vi "write_section_analysis_parameters_to_results_file.vi"(8 "Error In":errorcluster, 11 "Section Parameters":T1) -> (0 "Error Out":errorcluster)   [LabVIEW 2019]
uses:
  section_parameters_cluster_typedef.ctl
  sections_method_enum_typedef.ctl
  sections_edge_mode_enum_typedef.ctl
  sections_roi_size_enum_typedef.ctl
  xi_angles_enum_typedef.ctl
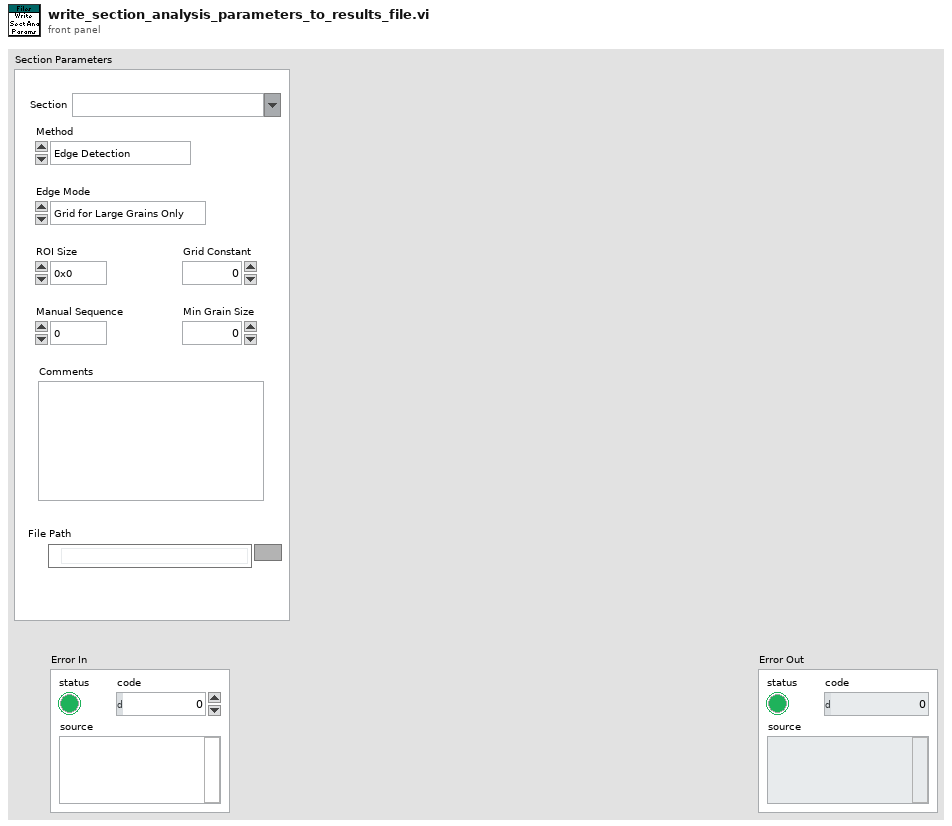
[diagram p1: front panel]
types:
  T1 = typedef "section_parameters_cluster_typedef.ctl" = cluster{"Section":string, "Method":T2, "Edge Mode":T3, "ROI Size":T4, "Manual Sequence":T5, "Grid Constant":i32, "Min Grain Size":dbl, "Comments":string, "File Path":path}
  T2 = typedef "sections_method_enum_typedef.ctl" = enum16{"Edge Detection", "Grid Only", "Manual Selection", "Existing Edges"}
  T3 = typedef "sections_edge_mode_enum_typedef.ctl" = enum16{"Grid for Large Grains Only", "Grid", "No Grid"}
  T4 = typedef "sections_roi_size_enum_typedef.ctl" = enum16{"0x0", "1x1", "2x2", "3x3", "4x4", "5x5", "6x6"}
  T5 = typedef "xi_angles_enum_typedef.ctl" = enum16{"0", "45"}
  T6 = typedef "writeable_section_parameters_cluster_typedef.ctl" = cluster{"Section":string, "Method":i32, "Edge Mode":i32, "Grid Constant":i32, "Manual Sequence":i32, "ROI Size":i32, "Min Grain Size":dbl, "Comments":string, "File Path":string}
  T7 = typedef "sample_results_cluster_typedef.ctl" = cluster{"File Path":string, "Sample":string, "Threshold":dbl, "Parameters":T8, "Writeable Parameters":T6, "Gain Results":T9[]}
  T8 = typedef "parameters_cluster_typedef.ctl" = cluster{"m1":dbl, "m2":dbl, "m3":dbl, "c":dbl, "D":dbl, "Beta":dbl, "center x":dbl, "center y":dbl}
  T9 = typedef "grain_results_cluster_typedef.ctl" = cluster{"Grain Number":i32, "xi":dbl[], "phiin":dbl[], "Intensity":dbl[][], "Best Fit Intensity":dbl[][], "Best Fit Parameters":dbl[][], "Polarizer 1 Angle":dbl[][], "Polarizer 2 Angle":dbl[][], "Best Extinction Angle":dbl[], "Best Extinction Angle Corrected":dbl[], "Thetac":dbl, "Phic":dbl, "ROI":cluster{"Global Rectangle":i32[], "Contours":cluster{"Contour Type":u32, "ROI Type":u32, "Points":i32[]}[]}, "a":dbl, "b":dbl, "sequences available":dbl, "sequences used":dbl, "Contrast":dbl[], "Rsq":dbl}
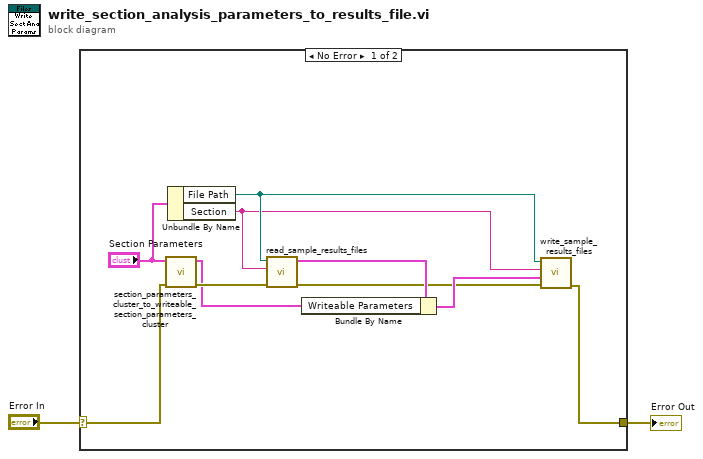
[diagram p0: block diagram]
diagram:
  n1 = case shown="No Error" "Error In" {
    selector: "Error In" -> [w12 w13]
    tunnel: [w3 w13] -> w1
    frame No Error {
      n2 = call "section_parameters_cluster_to_writeable_section_parameters_cluster.vi"("Error In"=w12, "Section Parameters"="Section Parameters") -> ("Error Out"=w11:errorcluster, "Writeable Parameters"=w8:T6)  [unwired: 8 in]
      n3 = Unbundle By Name("Section Parameters") -> ("File Path"=w5:path, "Section"=w4:string)
      n4 = call "read_sample_results_files.vi"("Error In"=w11, "Sample"=w4, "File Path"=w5) -> ("Error Out"=w6:errorcluster, "Sample Results"=w9:T7)  [unwired: 7 in]
      n5 = Bundle By Name(cluster=w9, "Writeable Parameters"=w8) -> (w7:T7)
      n6 = call "write_sample_results_files.vi"("Error In"=w6, "Sample Results"=w7, "Sample"=w4, "File Path"=w5) -> ("Error Out"=w3:errorcluster)  [unwired: 7 in]
    }
    frame Error {
    }
  }
  "Error Out" <- w1
